vi "SetExternalInterfaces.vi"(8 "ErrorIn":errorcluster, 10 "ExternalInterfaces":T1[](array[typedef]), 11 "ReferenceIn":refnum<class "MasterGUI.lvclass">) -> (0 "ErrorOut":errorcluster, 3 "ReferenceOut":refnum<class "MasterGUI.lvclass">)   [LabVIEW 2021, in "MasterGUI.lvclass"]
uses:
  MasterGUI.lvclass
  Library_TAF_Support/ClusterArrayConversion/BundledArray.ctl
  0a6ec689-4898-488c-8e07-ed5616c8d135.vi
  23b01655-c9ef-4a3c-a018-7f9b77e1bca9.vi
  Library_TAF_Support/ClusterArrayConversion/ClusterArrayConversion.lvlib
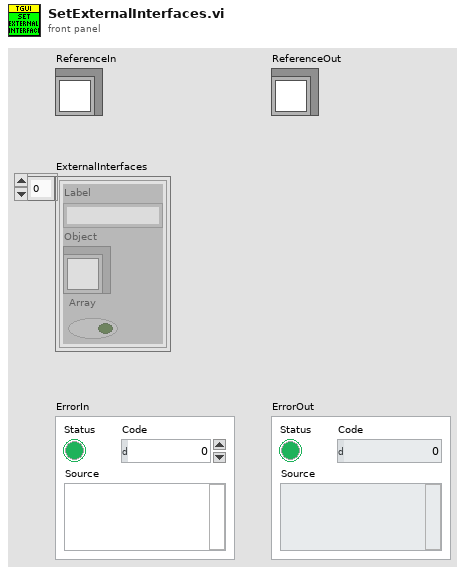
[diagram p1: front panel]
types:
  T1 = typedef "ClusterArrayConversion.lvlib/BundledArray.ctl" = cluster{"Label":string, "Object":refnum<class>, "Array":bool}
  T2 = typedef "MasterGUI.lvclass/ObjectAttributes.ctl" = cluster{"Interfaces":cluster{"Dummy":refnum<class>}, "Locals":cluster{"MainGUIActive":refnum<queue>, "MainPanel":refnum<vi>, "LayoutPanel":cluster{"PanelVIRef":refnum<vi>, "Labels":string[], "SubPanels":refnum<vi>[]}, "MenuTree":T3[], "Menu":refnum<k9>}, "Persistent":cluster{"StaticDocking":cluster{"ObjectLabel":string, "SubPanelLabel":string}[], "WindowsTitle":string, "AdditionalMenuItems":T3[], "TraceObjectName":string}}
  T3 = typedef "MasterGUI.lvclass/MenuItem.ctl" = cluster{"Parent":string, "Items":string[], "ShortCuts":cluster{"IncludeShiftKey":bool, "IncludeCtrlKey":bool, "ShortcutKey":string}[]}
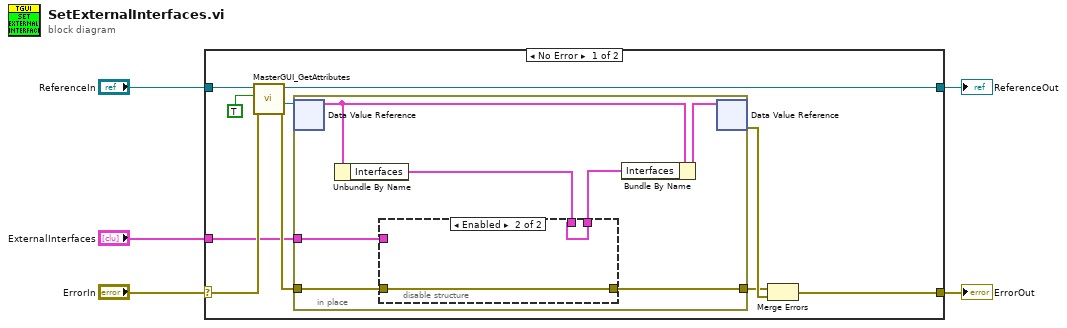
[diagram p0: block diagram]
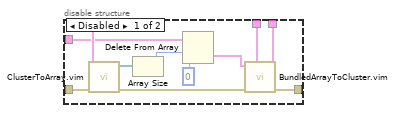
[diagram p2: hidden frame]
diagram:
  n1 = case shown="No Error" "ErrorIn" {
    selector: "ErrorIn" -> [w15 w36]
    tunnel: [w11 w36] -> w4
    tunnel: [w6 w35] -> w2
    tunnel: "ReferenceIn" -> [w10 w35]
    tunnel: "ExternalInterfaces" -> [w7 _]
    frame No Error {
      n2 = call "MasterGUI_GetAttributes.vi"("ErrorIn"=w15, "OnlyGetDvrReference(False)"=TRUE, "ReferenceIn"=w10) -> ("ErrorOut"=w12:errorcluster, "DataRef"=w8:refnum<data-value>, "ReferenceOut"=w6:refnum<class "MasterGUI.lvclass">)  [unwired: 5 in, 1 out]
      n3 = in-place {
        in-place-border: [w22] -> w13
        in-place-border: w12 -> [w21]
        in-place-border: w7 -> [w16]
        n4 = in-place-dvr #1(w8) -> (w19:T2)  [unwired: 1 out]
        n5 = Unbundle By Name(w19) -> ("Interfaces"=w17:cluster{"Dummy":refnum<class>})
        n6 = disable-structure shown="Enabled" {
          disable-tunnel: [w32 w34] -> w22
          disable-tunnel: [w29 w33] -> w18
          disable-tunnel: w17 -> [w28 w33]
          disable-tunnel: w16 -> [w27 _]
          disable-tunnel: w21 -> [w31 w34]
          frame Disabled {
            n7 = call "ClusterToArray.vim"("ErrorIn"=w31, "Cluster"=w28) -> ("ErrorOut"=w30:errorcluster, "ArrayOfElements"=w25:refnum<class>[])  [unwired: 7 in, 1 out]
            n8 = Array Size(array=w25) -> (size(s)=w24:i32)
            n9 = Delete From Array(array=w27, length=w24, index=0) -> (deleted portion=w26:T1[])  [unwired: 1 out]
            n10 = call "BundledArrayToCluster.vim"("Type"=w28, "ErrorIn"=w30, "BundeledLabels"=w26) -> ("ErrorOut"=w32:errorcluster, "DataOut"=w29:cluster{"Dummy":refnum<class>})  [unwired: 7 in]
          }
          frame Enabled {
          }
        }
        n11 = Bundle By Name(cluster=w19, "Interfaces"=w18) -> (w20:T2)
        n12 = in-place-dvr #1(w20) -> (w14:errorcluster)  [unwired: 1 out]
      }
      n13 = Merge Errors(w13, w14) -> (w11:errorcluster)
    }
    frame Error {
    }
  }
  "ErrorOut" <- w4
  "ReferenceOut" <- w2
